vi "Test_scale_champ.vi"() -> ()   [LabVIEW 2010]
panel:
  out "width":i32
  out "height":i32
  in  "path":path
  out "TableXYPos":cluster{dbl[], dbl[]}[](graph)=[{[-6.0, -6.0, 6.0, 6.0, -6.0], [-6.0, 6.0, 6.0, -6.0, -6.0]}, {[-24.087532979284084, 18.91195817688408], [-10.534566293522829, 14.291201500507801]}, {array[201 elements], array[201 elements]}, {[], []}, {[], []}, {[41.41679615624384, -5.804797830829483], [-35.677749550137705, -62.94114955013771]}, {[41.41679615624384, 14.153396156243835, -33.06819783082949, -5.804797830829483], [-35.677749550137705, 11.543844436935625, -15.719555563064382, -62.94114955013771]}]
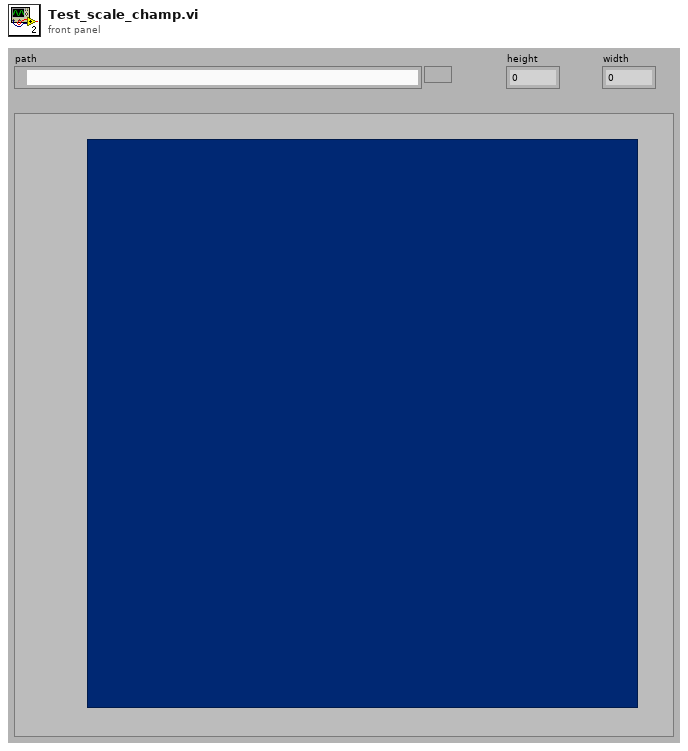
[diagram p1: front panel]
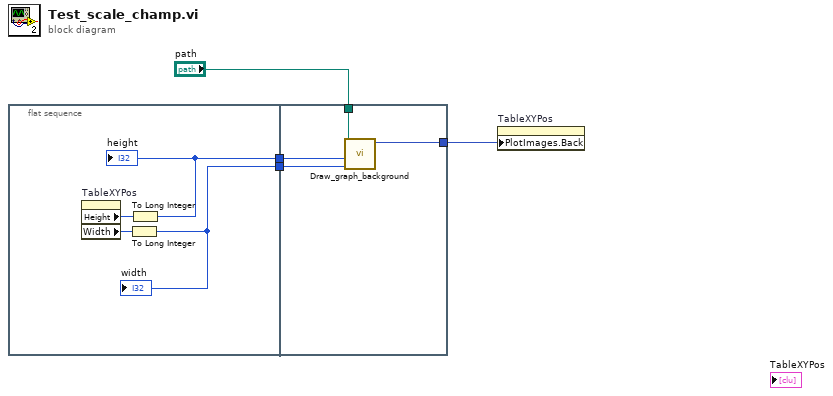
[diagram p0: block diagram]
diagram:
  n1 = flat-sequence {
    tunnel: [w6] -> w2
    tunnel: [w5] -> w1
    tunnel: "path" -> [w12]
    tunnel: [w11] -> w3
    tunnel: w2 -> [w10]
    tunnel: w1 -> [w9]
    frame #0 {
      n2 = property on="TableXYPos" class="XYGraph (strict)"() -> ("Height"=w8:u32, "Width"=w7:u32)  [unwired: 2 in, 2 out]
      n3 = To Long Integer(number=w7) -> (32bit integer=w5:i32)
      "width" <- w5
      n4 = To Long Integer(number=w8) -> (32bit integer=w6:i32)
      "height" <- w6
    }
    frame #1 {
      n5 = call "Draw_graph_background.vi"("New Width"=w9, "New Height"=w10, "path"=w12) -> ("Images"=w11:picture)  [unwired: 8 in]
    }
  }
  n6 = property on="TableXYPos" class="XYGraph (strict)"("PlotImages.Back"=w3) -> ()  [unwired: 2 in, 2 out]
